vi "tokenize string.vi"(10 "delimiter":string="/", 11 "raw path":string) -> (3 "segments":string[](array[string]))   [LabVIEW 2013, in "uniform resource locator.lvlib"]
uses:
  uniform resource locator.lvlib
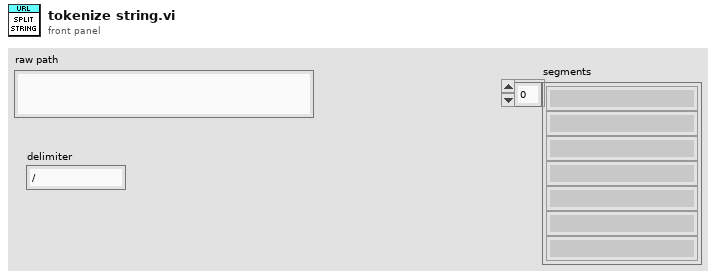
[diagram p1: front panel]
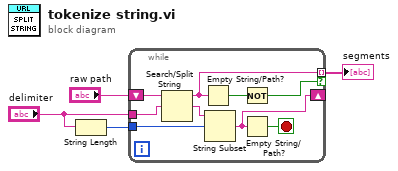
[diagram p0: block diagram]
diagram:
  n1 = String Length(string="delimiter") -> (length=w1:i32)
  n2 = while {
    shift-right: [w11] -> _
    shift-left: "raw path" -> [w13]
    tunnel: [w7] -> w3 mode=indexing if=w5
    tunnel: "delimiter" -> [w9]
    tunnel: w1 -> [w8]
    stop <- w10 stop-if-true
    n3 = Search/Split String(string=w13, search string/char (-)=w9) -> (substring before match=w7:string, match + rest of string=w12:string)  [unwired: 1 in, 1 out]
    n4 = Empty String/Path?(string/path=w7) -> (empty?=w6:bool)
    n5 = String Subset(string=w12, offset (0)=w8) -> (substring=w11:string)  [unwired: 1 in]
    n6 = Not(x=w6) -> (.not. x?=w5:bool)
    n7 = Empty String/Path?(string/path=w11) -> (empty?=w10:bool)
  }
  "segments" <- w3
